vi "Get Service Class Instances.vi"() -> (3 "service instances":refnum<class "ServiceBase.lvclass">[](array[class]))   [LabVIEW 2025, in "calculator_server.lvlib"]
uses:
  calculator_server.lvlib
  <vilib>/gRPC/LabVIEW gRPC Servicer/ServiceBase/ServiceBase.lvclass
  RPC Service/Calculator/Calculator.lvclass
  C:/Program Files/National Instruments/LabVIEW 2025/vi.lib/gRPC/LabVIEW gRPC Servicer/ServiceBase/ServiceBase.lvclass
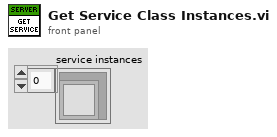
[diagram p1: front panel]
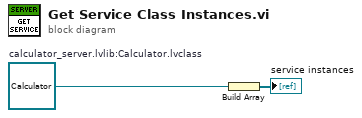
[diagram p0: block diagram]
diagram:
  w1 = refnum<class "Calculator.lvclass"> refnum  # calculator_server.lvlib:Calculator.lvclass
  n1 = Build Array(w1) -> (→"service instances":refnum<class "Calculator.lvclass">[])
